vi "UTIL_retrieve_resource v1_0_0.vi"(8 "error in":T1, 9 "Display Dialog On Error":bool=TRUE, 10 "Resources":string[](array[string]), 11 "Resource Name":string) -> (0 "error out":T1, 1 "Resource String":string, 2 "Resource Number":dbl format="%.3f", 3 "Resource Integer":i32)   [LabVIEW 2015]
doc: "UTIL_retrieve_resource v1_0_0.vi\n\nThis VI looks for a match in the Global RM Resource variable for a given name. If it is found the associated value is returned. If the name is NOT found an error is show with a dialog box.\n\nResource Name: the name of the resource.\n\nDisplay Dialog On Error: if TRUE a dialog box will display an error condition. If FALSE on box is shown. Default is TRUE.\n\nResource Integer: the integer value.\n\nResource Number: the real number value.\n\nResource String: the string value.\n\nerror out: a error cluster. The cluster contains a boolean, error code and string. The boolean indicates if an error occured, the code is -1 on error and 0 for no error and the string contains the resource name that can not be found."
panel:
  # "TRUE"
  # "FALSE"
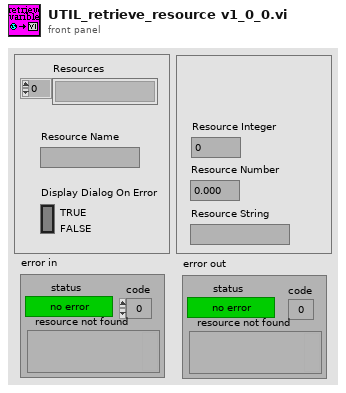
[diagram p1: front panel]
types:
  T1 = cluster{"status":bool, "code":i32, "resource not found":string}
  T2 = cluster{"status":bool, "code":i32, "Resource Name":string}
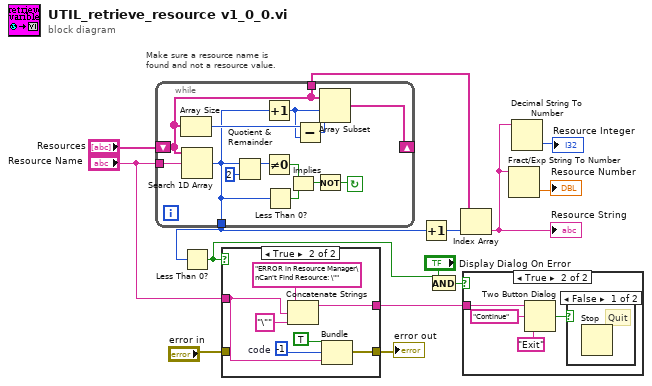
[diagram p0: block diagram]
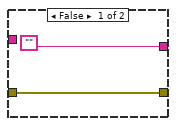
[diagram p4: hidden frame]
diagram:
  # "Make sure a resource name is found and not a resource value."
  n1 = while {
    tunnel: [w20] -> w3
    shift-left: "Resources" -> [w20]
    shift-right: [w24] -> _
    tunnel: [w19] -> w4
    tunnel: "Resource Name" -> [w27]
    stop <- w15 continue-if-true
    n2 = Array Size(array=w20) -> (size(s)=w23:i32)
    n3 = Search 1D Array(1D array=w20, element=w27) -> (index of element=w19:i32)  [unwired: 1 out]
    n4 = Quotient & Remainder(x=w19, y=2) -> (x-y*floor(x/y)=w25:i32)  [unwired: 1 out]
    n5 = Increment(x=w19) -> (x+1=w22:i32)
    n6 = Not Equal To 0?(x=w25) -> (x != 0?=w18:bool)
    n7 = Less Than 0?(x=w19) -> (x < 0?=w17:bool)
    n8 = Implies(1:w17, 2:w18) -> (0:w16:bool)
    n9 = Subtract(x=w23, y=w22) -> (x-y=w21:i32)
    n10 = Not(x=w16) -> (.not. x?=w15:bool)
    n11 = Array Subset(array=w20, index=w22, length=w21) -> (w24:string[])
  }
  n12 = Less Than 0?(x=w4) -> (x < 0?=w8:bool)
  n13 = case shown="True" w8 {
    tunnel: "Resource Name" -> [_ w31]
    tunnel: [w28 w30] -> w5
    tunnel: ["" w34] -> w9
    tunnel: "error in" -> [w28 _]
    frame False {
    }
    frame True {
      w32 = -1  # code
      n14 = Concatenate Strings("ERROR in Resource Manager\nCan't Find Resource: \"", w31, "\"" ("Resource Name")) -> (w34:string)
      n15 = Bundle("status"=TRUE, "code"=w32, "Resource Name"=w31) -> (w30:T2)  [unwired: 1 out]
    }
  }
  "error out" <- w5
  n16 = Increment(x=w4) -> (x+1=w13:i32)
  n17 = And(x="Display Dialog On Error", y=w8) -> (x .and. y?=w6:bool)
  n18 = Index Array(array=w3, index=w13) -> (element=w11:string)
  "Resource String" <- w11
  n19 = case shown="True" w6 {
    tunnel: w9 -> [_ w40]
    frame False {
    }
    frame True {
      n20 = Two Button Dialog(message=w40, 1:"Exit" ("F button name (\"Cancel\")"), 2:"Continue" ("T button name (\"OK\")")) -> (T button?=w39:bool)
      n21 = case shown="False" w39 {
        frame False {
          # "Quit"
          n22 = Stop() -> ()  [unwired: 1 out]
        }
        frame True {
        }
      }
    }
  }
  n23 = Fract/Exp String To Number(string=w11) -> (number=→"Resource Number":dbl)  [unwired: 4 out]
  n24 = Decimal String To Number(string=w11) -> (number=→"Resource Integer":i32)  [unwired: 3 out]
